vi "Aperture status converter.vi"(11 "Aperture Position":cluster{"IN sensor":bool, "OUT sensor":bool}) -> (3 "Aperture Status":T1)   [LabVIEW 2016]
doc: "Converts position sensor data to a state:\nAperture in (IN sensor = TRUE; OUT sensor = FALSE)\nAperture out (IN sensor = FALSE; OUT sensor = TRUE)\nAperture status unclear (IN sensor = OUT sensor)"
uses:
  Aperture states.ctl
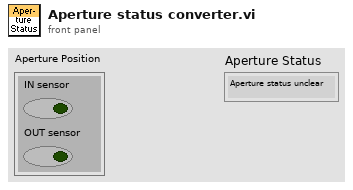
[diagram p1: front panel]
types:
  T1 = typedef "Aperture states.ctl" = enum16{"Aperture status unclear", "Aperture in", "Aperture out"}
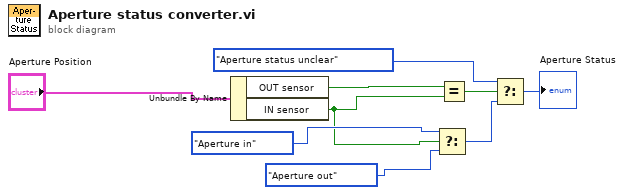
[diagram p0: block diagram]
diagram:
  n1 = Unbundle By Name("Aperture Position") -> ("OUT sensor"=w4:bool, "IN sensor"=w2:bool)
  n2 = Select(t=Aperture_states."Aperture in" ("Enum"), s=w2, f=Aperture_states."Aperture out" ("Enum")) -> (s? t:f=w1:T1)
  n3 = Equal?(x=w4, y=w2) -> (x = y?=w3:bool)
  n4 = Select(t=Aperture_states."Aperture status unclear" ("Enum"), s=w3, f=w1) -> (s? t:f=→"Aperture Status":T1)
